vi "FG_FPGA_Interface_Servo.vi"(7 "Action":T1, 8 "error in":errorcluster) -> (0 "error out":errorcluster, 3 "FPGA VI Reference Out":refnum<k20>)   [LabVIEW 2014]
uses:
  Typedef_FPGA_Interface_Action.ctl
  <vilib>/FPGAPlugInAG/sbRIO-9626/niLvFpga_Open_sbRIO-9626.vi
  <vilib>/rvi/interface/common/dynamic/niFpgaDynamicAddResources.vi
  <vilib>/nisyscfg/Initialize (Control).vi
  <vilib>/nisyscfg/Find Hardware.vi
  <vilib>/Utility/error.llb/Error Cluster From Error Code.vi
  <vilib>/rvi/errors/niLvFpgaAdjustHostInterfaceError.vi
  <vilib>/FPGAPlugInAG/Dynamic/niLvFpga_Close_Dynamic.vi
  <vilib>/rvi/interface/nirviOpenFPGA/nirviOpenFPGA.xnode
  FPGA Bitfiles/Main FPGA 5-axis Servo.lvbitx
  <vilib>/rvi/interface/nirviReadWriteControl/nirviReadWriteControl.xnode
  <vilib>/rvi/interface/nirviCloseFPGA/nirviCloseFPGA.xnode
  <vilib>/nisyscfg/nisyscfg.lvlib
  NiFpgaLv.dll
  <vilib>/rvi/interface/Simulation/niFpgaSimulationCallBeginRW.vi
panel:
  out "Numeric":i32
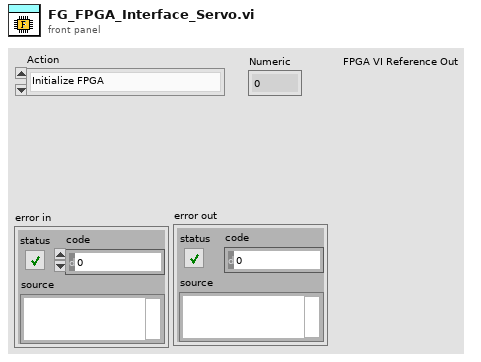
[diagram p1: front panel]
types:
  T1 = typedef "Typedef_FPGA_Interface_Action.ctl" = enum16{"Initialize FPGA", "Get FPGA Reference", "Close FPGA"}
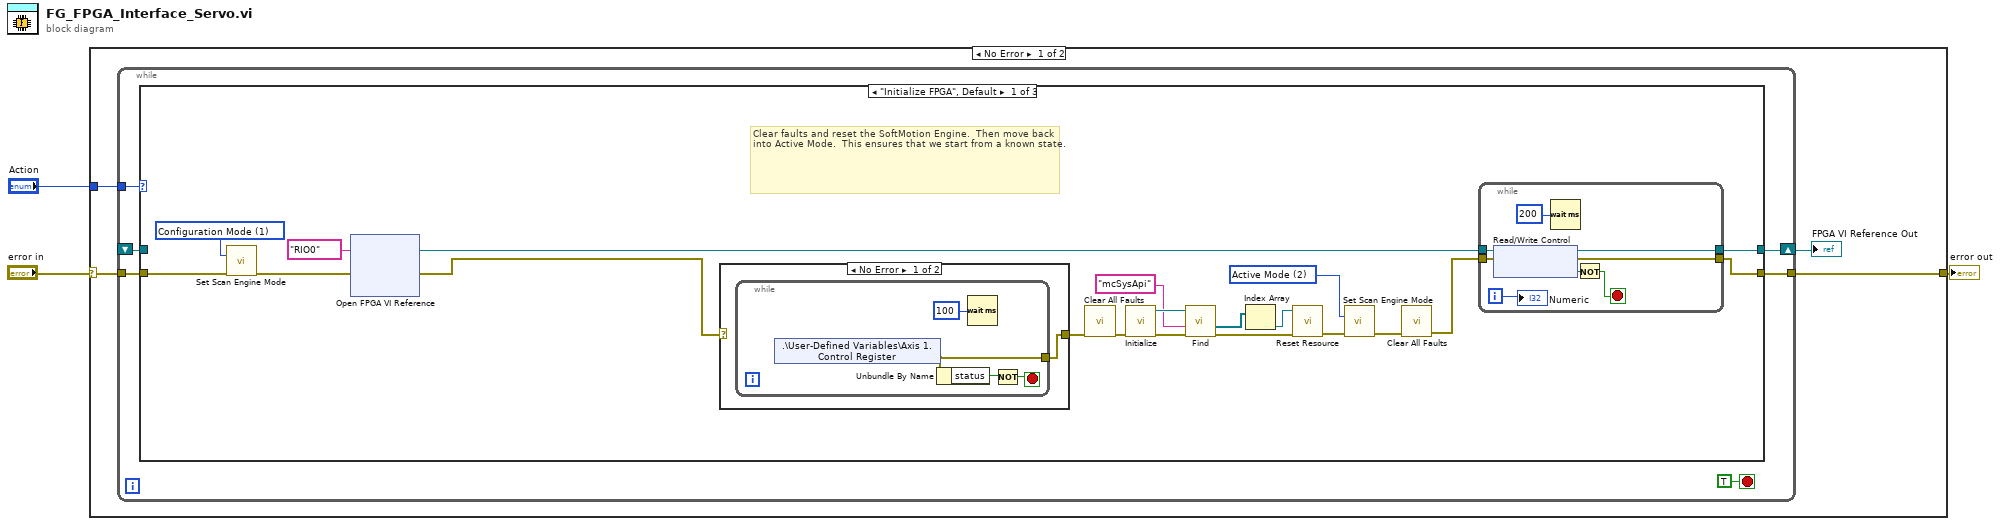
[diagram p0: block diagram]
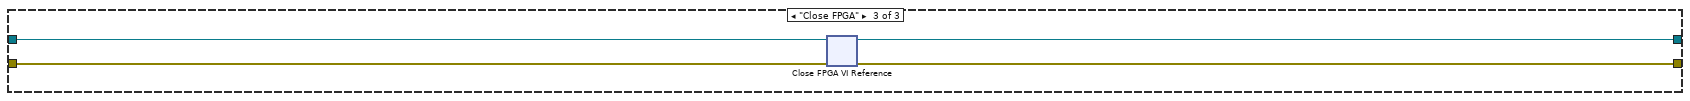
[diagram p4: hidden frame]
diagram:
  n1 = case shown="No Error" "error in" {
    selector: "error in" -> [w7 w53]
    tunnel: [w6 w53] -> w2
    tunnel: "Action" -> [w5 _]
    frame No Error {
      n2 = while {
        tunnel: w7 -> [w11]
        tunnel: w5 -> [w12]
        tunnel: [w10] -> w6
        shift-right: [w9] -> w4
        shift-left: _ -> [w8]
        stop <- TRUE stop-if-true
        n3 = case shown="\"Initialize FPGA\", Default" w12 {
          tunnel: w11 -> [w32 w48 w51]
          tunnel: [w19 w48 w52] -> w10
          tunnel: w8 -> [_ w49 w50]
          tunnel: [w20 w49 w50] -> w9
          frame "Initialize FPGA", Default {
            w21 = 2 items=["Configuration Mode"=1, "Active Mode"=2] ("mode (Active Mode)")
            w29 = 1 items=["Configuration Mode"=1, "Active Mode"=2] ("mode (Active Mode)")
            # "Clear faults and reset the SoftMotion Engine.  Then move back into Active Mode.  This ensures that we start from a known state."
            n4 = call <vilib>:"Set Scan Engine Mode.vi"("mode (Active Mode)"=w29, "error in (no error)"=w32) -> ("error out"=w31:errorcluster)  [unwired: 13 in]
            n5 = xnode "Open FPGA VI Reference"("error in"=w31, "resource name"=tag "RIO0") -> ("FPGA VI Reference Out"=w14:refnum<k20>, "error out"=w15:errorcluster)
            n6 = case shown="No Error" w15 {
              selector: w15 -> [_ w47]
              tunnel: [w42 w47] -> w30
              frame No Error {
                n7 = while {
                  tunnel: [w43] -> w42
                  stop <- w46 stop-if-true
                  n8 = shared-variable ".\\User-Defined Variables\\Axis 1.Control Register"() -> (error out=w43:errorcluster)  [unwired: 1 in, 1 out]
                  n9 = Unbundle By Name(w43) -> ("status"=w45:bool)
                  n10 = Wait (ms)(milliseconds to wait=u32 100) -> ()  [unwired: 1 out]
                  n11 = Not(x=w45) -> (.not. x?=w46:bool)
                }
              }
              frame Error {
              }
            }
            n12 = call <vilib>:"Clear All Faults.vi"("error in (no error)"=w30) -> ("error out"=w28:errorcluster)  [unwired: 10 in]
            n13 = call-poly <vilib>:"Initialize.vi"("error in (no error)"=w28) -> ("error out"=w22:errorcluster, "Session out"=w24:refnum<k21>)  [unwired: 8 in, 1 out]
            n14 = call-poly <vilib>:"Find.vi"("error in (no error)"=w22, "Experts"="mcSysApi" ("experts"), "Session in"=w24) -> ("error out"=w27:errorcluster, "Resources out"=w25:refnum<k20>[])  [unwired: 5 in, 2 out]
            n15 = Index Array(array=w25) -> (element=w26:refnum<k20>)  [unwired: 1 in]
            n16 = call <vilib>:"Reset Resource.vi"("error in (no error)"=w27, "Resource in"=w26) -> ("error out"=w18:errorcluster)  [unwired: 8 in, 1 out]
            n17 = call <vilib>:"Set Scan Engine Mode.vi"("mode (Active Mode)"=w21, "error in (no error)"=w18) -> ("error out"=w17:errorcluster)  [unwired: 13 in]
            n18 = call <vilib>:"Clear All Faults.vi"("error in (no error)"=w17) -> ("error out"=w16:errorcluster)  [unwired: 10 in]
            n19 = while {
              tunnel: w16 -> [w41]
              tunnel: [w40] -> w19
              tunnel: w14 -> [w36]
              tunnel: [w35] -> w20
              i -> [w34]
              stop <- w37 stop-if-true
              n20 = xnode "Read/Write Control"("FPGA VI Reference In"=w36, "error in"=w41) -> ("FPGA VI Reference Out"=w35:refnum<k20>, "error out"=w40:errorcluster, "Sync is Fault"=w39:bool)
              n21 = Wait (ms)(milliseconds to wait=u32 200) -> ()  [unwired: 1 out]
              n22 = Not(x=w39) -> (.not. x?=w37:bool)
              "Numeric" <- w34
            }
          }
          frame "Get FPGA Reference" {
          }
          frame "Close FPGA" {
            n23 = xnode "Close FPGA VI Reference"("FPGA VI Reference In"=w50, "error in"=w51) -> ("error out"=w52:errorcluster)
          }
        }
      }
      "FPGA VI Reference Out" <- w4
    }
    frame Error {
    }
  }
  "error out" <- w2
